vi "PacketToLoggingData.vi"(0 "PacketArray":T1[](array[typedef])) -> (4 "Array 6":i16[][](array[numeric]), 6 "Latitude":sgl[](array[numeric]), 8 "Longittude":sgl[](array[numeric]), 15 "LoggingData":sgl[](array[numeric]))   [LabVIEW 2023]
uses:
  controls/glbRoboterData.ctl
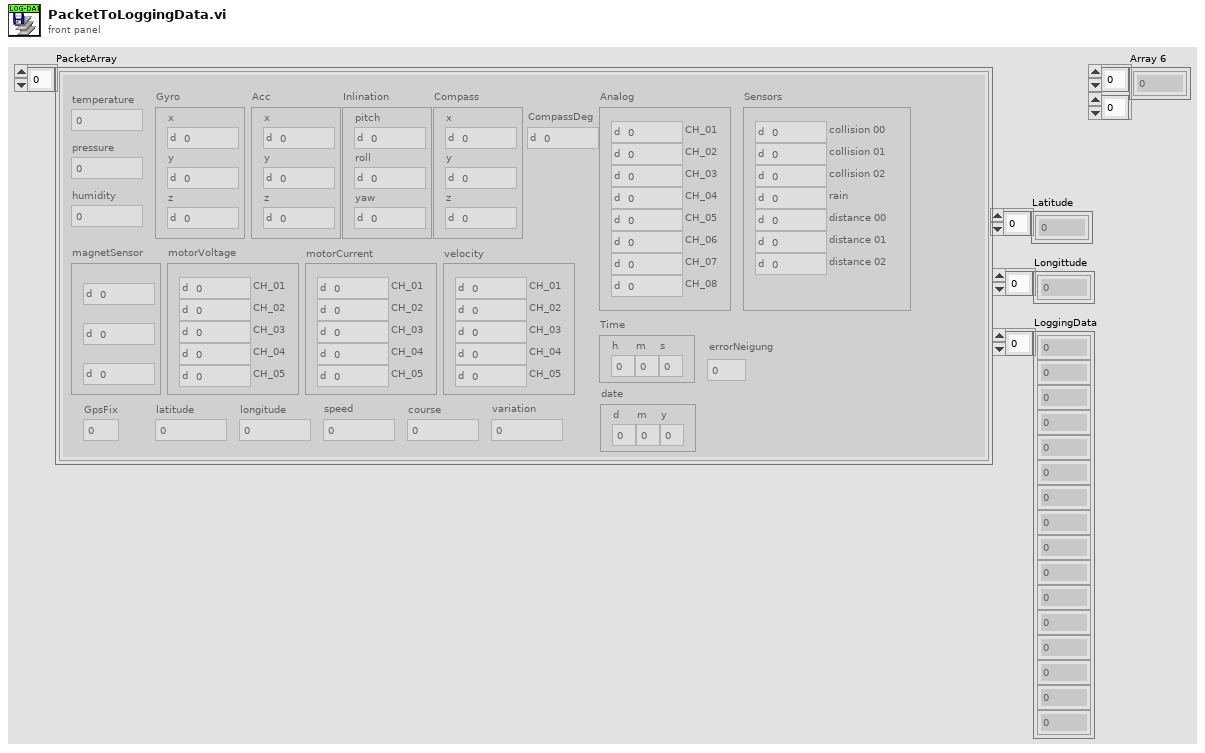
[diagram p1: front panel]
types:
  T1 = typedef "glbRoboterData.ctl" = cluster{"temperature":i16, "pressure":i16, "humidity":i16, "Gyro":cluster{"x":i16, "y":i16, "z":i16}, "Acc":cluster{"x":i16, "y":i16, "z":i16}, "Inlination":cluster{"pitch":i16, "roll":i16, "yaw":i16}, "Compass":cluster{"x":i16, "y":i16, "z":i16}, "CompassDeg":u32, "Analog":cluster{"CH_01":i16, "CH_02":i16, "CH_03":i16, "CH_04":i16, "CH_05":i16, "CH_06":i16, "CH_07":i16, "CH_08":i16}, "magnetSensor":cluster{"x":i16, "y":i16, "z":i16}, "motorVoltage":cluster{"CH_01":i16, "CH_02":i16, "CH_03":i16, "CH_04":i16, "CH_05":i16}, "motorCurrent":cluster{"CH_01":i16, "CH_02":i16, "CH_03":i16, "CH_04":i16, "CH_05":i16}, "velocity":cluster{"CH_01":i16, "CH_02":i16, "CH_03":i16, "CH_04":i16, "CH_05":i16}, "GpsFix":u8, "latitude":sgl, "longitude":sgl, "speed":sgl, "course":sgl, "variation":sgl, "Time":cluster{"h":u8, "m":u8, "s":u8}, "date":cluster{"d":u8, "m":u8, "y":u8}, "errorNeigung":i8, "Sensors":cluster{"collision 00":u8, "collision 01":u8, "collision 02":u8, "rain":u16, "distance 00":u16, "distance 01":u16, "distance 02":u16}}
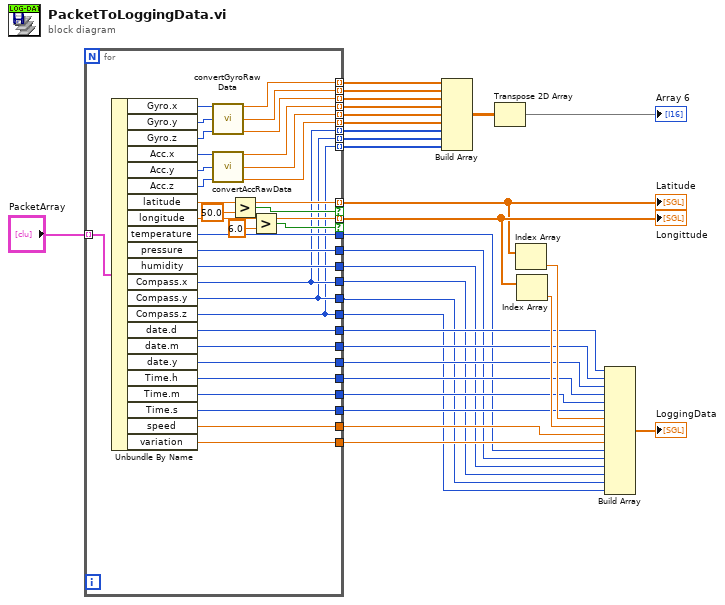
[diagram p0: block diagram]
diagram:
  n1 = for {
    tunnel: "PacketArray" -> [w64] mode=indexing
    tunnel: [w36] -> w21 mode=indexing
    tunnel: [w35] -> w22 mode=indexing
    tunnel: [w34] -> w23 mode=indexing
    tunnel: [w40] -> w24 mode=indexing
    tunnel: [w39] -> w25 mode=indexing
    tunnel: [w38] -> w26 mode=indexing
    tunnel: [w60] -> w12 mode=indexing if=w57
    tunnel: [w59] -> w19 mode=indexing if=w58
    tunnel: [w63] -> w9
    tunnel: [w62] -> w8
    tunnel: [w61] -> w7
    tunnel: [w46] -> w6
    tunnel: [w45] -> w5
    tunnel: [w44] -> w4
    tunnel: [w54] -> w18
    tunnel: [w53] -> w17
    tunnel: [w52] -> w16
    tunnel: [w51] -> w15
    tunnel: [w50] -> w14
    tunnel: [w49] -> w13
    tunnel: [w48] -> w11
    tunnel: [w47] -> w10
    tunnel: [w46] -> w3 mode=indexing
    tunnel: [w45] -> w2 mode=indexing
    tunnel: [w44] -> w1 mode=indexing
    n2 = Unbundle By Name(w64) -> ("Gyro.x"=w37:i16, "Gyro.y"=w33:i16, "Gyro.z"=w32:i16, "Acc.x"=w43:i16, "Acc.y"=w42:i16, "Acc.z"=w41:i16, "latitude"=w60:sgl, "longitude"=w59:sgl, "temperature"=w63:i16, "pressure"=w62:i16, "humidity"=w61:i16, "Compass.x"=w46:i16, "Compass.y"=w45:i16, "Compass.z"=w44:i16, "date.d"=w54:u8, "date.m"=w53:u8, "date.y"=w52:u8, "Time.h"=w51:u8, "Time.m"=w50:u8, "Time.s"=w49:u8, "speed"=w48:sgl, "variation"=w47:sgl)
    n3 = call "convertGyroRawData.vi"("raw x"=w37, "raw y"=w33, "raw z"=w32) -> ("x"=w36:sgl, "y"=w35:sgl, "z"=w34:sgl)  [unwired: 10 in]
    n4 = call "convertAccRawData.vi"("raw x"=w43, "raw y"=w42, "raw z"=w41) -> ("x"=w40:sgl, "y"=w39:sgl, "z"=w38:sgl)  [unwired: 10 in]
    n5 = Greater?(x=w60, y=sgl 50.0 ("x")) -> (0:w57:bool)
    n6 = Greater?(x=w59, y=sgl 6.0 ("x")) -> (0:w58:bool)
  }
  "Longittude" <- w19
  "Latitude" <- w12
  n7 = Build Array(w21, w22, w23, w24, w25, w26, w3, w2, w1) -> (w27:sgl[][])
  n8 = Transpose 2D Array(2D array=w27) -> (transposed array=→"Array 6":sgl[][])
  n9 = Index Array(array=w12) -> (element=w30:sgl)  [unwired: 1 in]
  n10 = Index Array(array=w19) -> (element=w31:sgl)  [unwired: 1 in]
  n11 = Build Array(w18, w17, w16, w15, w14, w13, w30, w31, w11, w10, w9, w8, w7, w6, w5, w4) -> (→"LoggingData":sgl[])
